vi "Receive UDP.vi"() -> (3 "Position":T1)   [LabVIEW 2011]
panel:
  in  "Numeric":dbl
  out "Cluster":cluster{"Numeric":dbl}
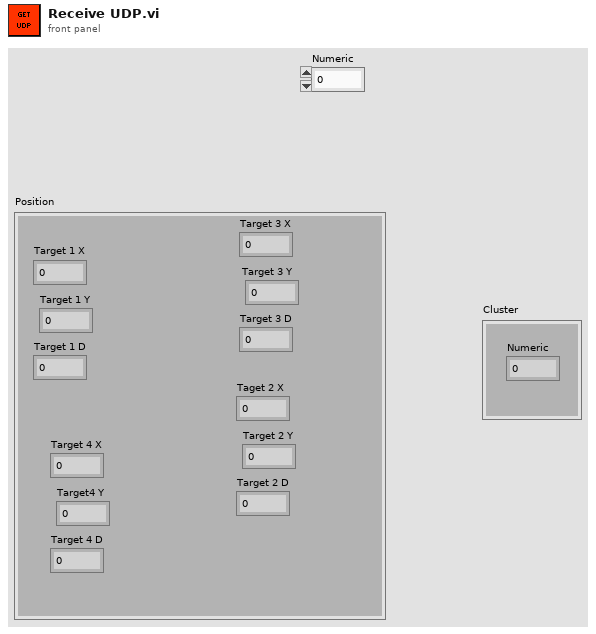
[diagram p1: front panel]
types:
  T1 = cluster{"Target 4 X":dbl, "Target4 Y":dbl, "Target 4 D":dbl, "Target 1 X":dbl, "Target 1 Y":dbl, "Target 1 D":dbl, "Target 3 X":dbl, "Target 3 Y":dbl, "Target 3 D":dbl, "Taget 2 X":dbl, "Target 2 Y":dbl, "Target 2 D":dbl}
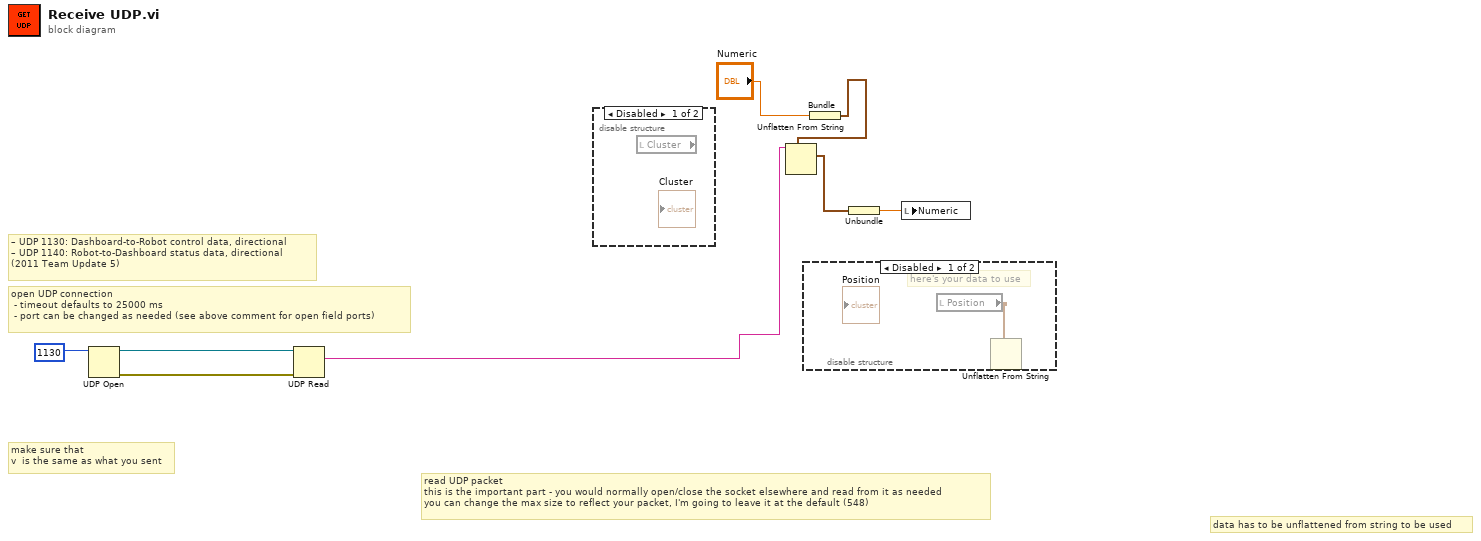
[diagram p0: block diagram]
diagram:
  # "make sure that\nv  is the same as what you sent"
  # "data has to be unflattened from string to be used"
  # "read UDP packet\nthis is the important part - you would normally open/close the socket elsewhere and read from it as needed\nyou can change the max size to reflect your packet, I'm going to leave it at the default (548)"
  # "open UDP connection\n - timeout defaults to 25000 ms\n - port can be changed as needed (see above comment for open field ports)"
  # "– UDP 1130: Dashboard-to-Robot control data, directional\n– UDP 1140: Robot-to-Dashboard status data, directional\n(2011 Team Update 5)"
  n1 = UDP Open(11:u16 1130 ("port")) -> (port=w7:refnum<k16>, 0:w6:errorcluster)  [unwired: 1 in, 4 out]
  n2 = UDP Read(connection ID=w7, 8:w6) -> (data out=w5:string)  [unwired: 6 out]
  n3 = disable-structure shown="Disabled" {
    frame Disabled {
      n4 = local read "Cluster"() -> ()  [unwired: 1 out]
    }
    frame Enabled {
    }
  }
  n5 = disable-structure shown="Disabled" {
    frame Disabled {
      # "here's your data to use"
      n6 = local read "Position"() -> (w9:T1)
      n7 = Unflatten From String(type=w9) -> ()  [unwired: 2 in, 5 out]
    }
    frame Enabled {
    }
  }
  n8 = Bundle("Numeric"="Numeric") -> (w3:cluster{"Numeric":dbl})  [unwired: 1 in]
  n9 = Unflatten From String(type=w3, binary string=w5) -> (value=w2:cluster{"Numeric":dbl})  [unwired: 1 in, 4 out]
  n10 = Unbundle(w2) -> ("Numeric"=w1:dbl)
  n11 = local write "Numeric"(w1) -> ()
